vi "synnax_client_smoke_test.vi"() -> ()   [LabVIEW 2026]
uses:
  lvlib/typedefs/connection_config.ctl
  lvlib/classes/Client/Private/synnax channel retrieve keys Array.vi
  lvlib/classes/Writer/Private/synnax writer open Array.vi
  lvlib/classes/Writer/Private/Writes/DBL/Write 1Ch NSamp (DBL).vi
  lvlib/classes/Synnax Writer.lvclass
  lvlib/classes/Client/Synnax Client.lvclass
  lvlib/synnax_clib.lvlib
panel:
  in  "names":string[](array[numeric])=["some_f64", "some_idx"]
  in  "Connection Config":T1={"host"="localhost", "port"=9090, "username"="synnax", "password"="seldon"}
  in  "Value":dbl=1.1
  out "error out":errorcluster
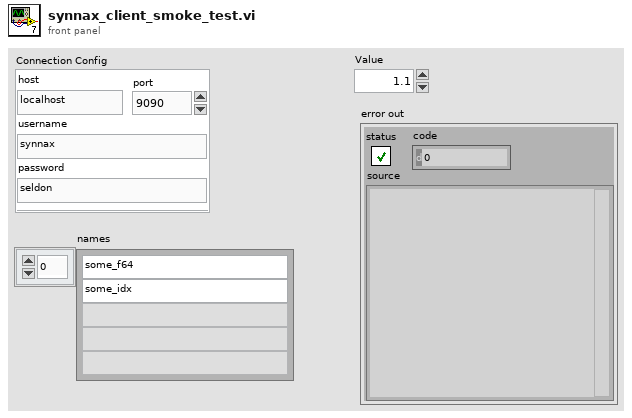
[diagram p1: front panel]
types:
  T1 = typedef "synnax_clib.lvlib/connection_config.ctl" = cluster{"host":string, "port":u16, "username":string, "password":string}
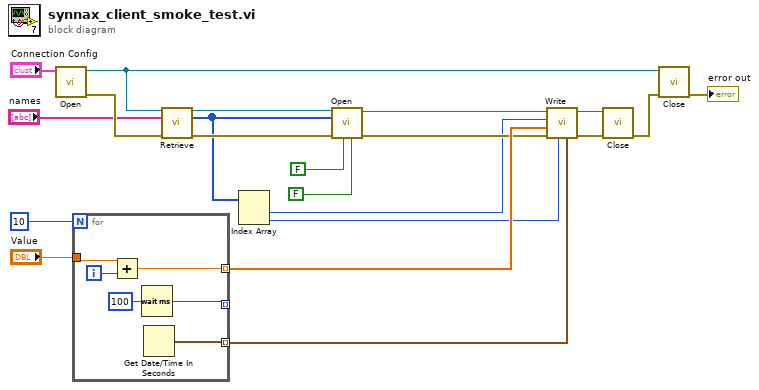
[diagram p0: block diagram]
diagram:
  n1 = call "Open.vi"("Connection Config"="Connection Config") -> ("error out"=w15:errorcluster, "Synnax Client out"=w18:refnum<class "Synnax Client.lvclass">)  [unwired: 9 in]
  n2 = for {
    N: 10 -> [_]
    tunnel: "Value" -> [w27]
    tunnel: [w25] -> w9 mode=indexing
    tunnel: [w24] -> _ mode=indexing
    tunnel: [w23] -> w7 mode=indexing
    i -> [w26]
    n3 = Add(x=w27, y=w26) -> (x+y=w25:dbl)
    n4 = Wait (ms)(milliseconds to wait=u32 100) -> (millisecond timer value=w24:u32)
    n5 = Get Date/Time In Seconds() -> (seconds since 1Jan1904=w23:timestamp)
  }
  n6 = call-poly "Retrieve.vi"("Synnax Client in"=w18, "names"="names", "error in"=w15) -> ("Synnax Client out"=w2:refnum<class "Synnax Client.lvclass">, "keys"=w1:u32[], "error out"=w20:errorcluster)  [unwired: 9 in, 1 out]
  n7 = Index Array(array=w1) -> (element #1=w3:u32, element #2=w4:u32)  [unwired: 2 in]
  n8 = call-poly "Open.vi"("enable_auto_commit (F)"=FALSE, "auto_index (F)"=FALSE, "error in"=w20, "channels in"=w1, "Synnax Client in"=w2) -> ("error out"=w8:errorcluster, "writer out"=w14:refnum<class "Synnax Writer.lvclass">)  [unwired: 4 in, 1 out]
  n9 = call-poly "Write.vi"("timestamps"=w7, "index_channel"=w4, "error in"=w8, "data"=w9, "channel"=w3, "Writer"=w14) -> ("error out"=w21:errorcluster, "Writer Out"=w13:refnum<class "Synnax Writer.lvclass">)  [unwired: 4 in]
  n10 = call "Close.vi"("error in"=w21, "writer"=w13) -> ("error out"=w17:errorcluster)  [unwired: 9 in]
  n11 = call "Close.vi"("error in"=w17, "Synnax Client in"=w18) -> ("error out"=→"error out":errorcluster)  [unwired: 9 in]
